vi "FRA-TEC.vi"(0 "LoadProcedure":refnum<k24>, 4 "stop":bool, 7 "error in":errorcluster) -> (18 "Bode phase":cluster{"Y":dbl[], "Y":dbl[]}[](graph), 19 "Bode Z":cluster{"Y":dbl[], "Y":dbl[]}[](graph), 20 "Nyquist":cluster{"Y":dbl[], "Y":dbl[]}[](graph), 21 "E & I":cluster{"Y":dbl[], "Y":dbl[]}[](graph), 22 "-Phase":dbl[](array[numeric]), 23 "Frequency":dbl[](array[numeric]), 24 "-Z''":dbl[](array[numeric]), 25 "Z":dbl[](array[numeric]), 26 "Z'":dbl[](array[numeric]), 27 "error out":errorcluster)   [LabVIEW 2014]
doc: "Shows the Frequency Response Analysis measured values from the instrument."
uses:
  C:/Users/user/Documents/Andre/AutoLAB-2017/Labview/Autolab SDK 1.11/EcoChemie.Autolab.Sdk.dll
  EcoChemie.Autolab.Sdk.dll
  Global 1.vi
  C:/Users/user/Documents/Andre/AutoLAB-2017/Labview/Autolab SDK 1.11/EcoChemie100.dll
  EcoChemie100.dll
panel:
  out "Event":bool
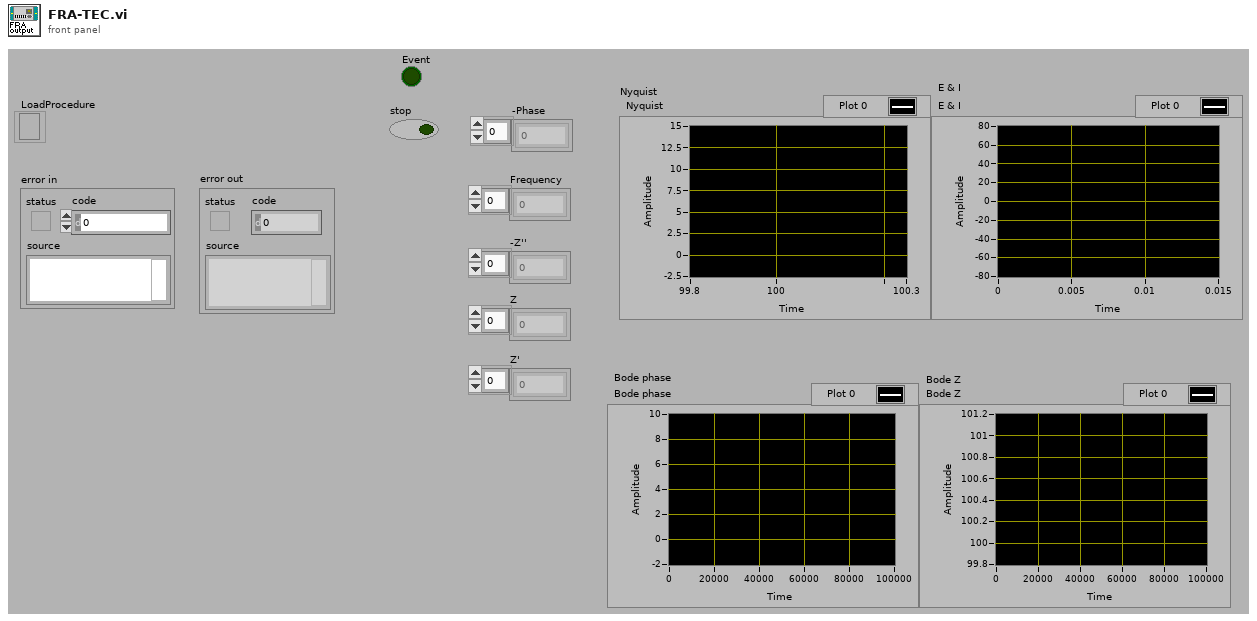
[diagram p1: front panel]
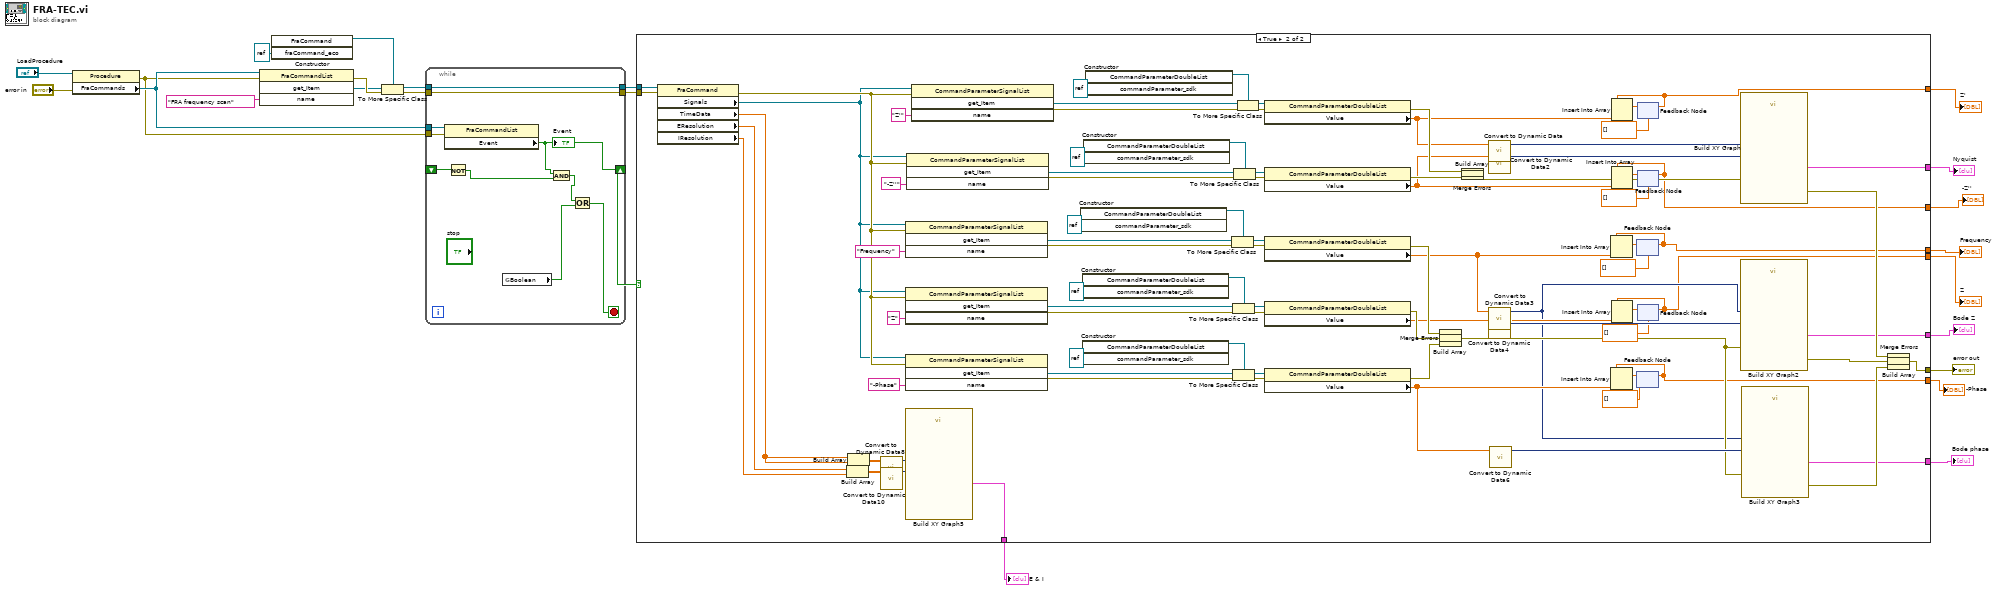
[diagram p0: block diagram]
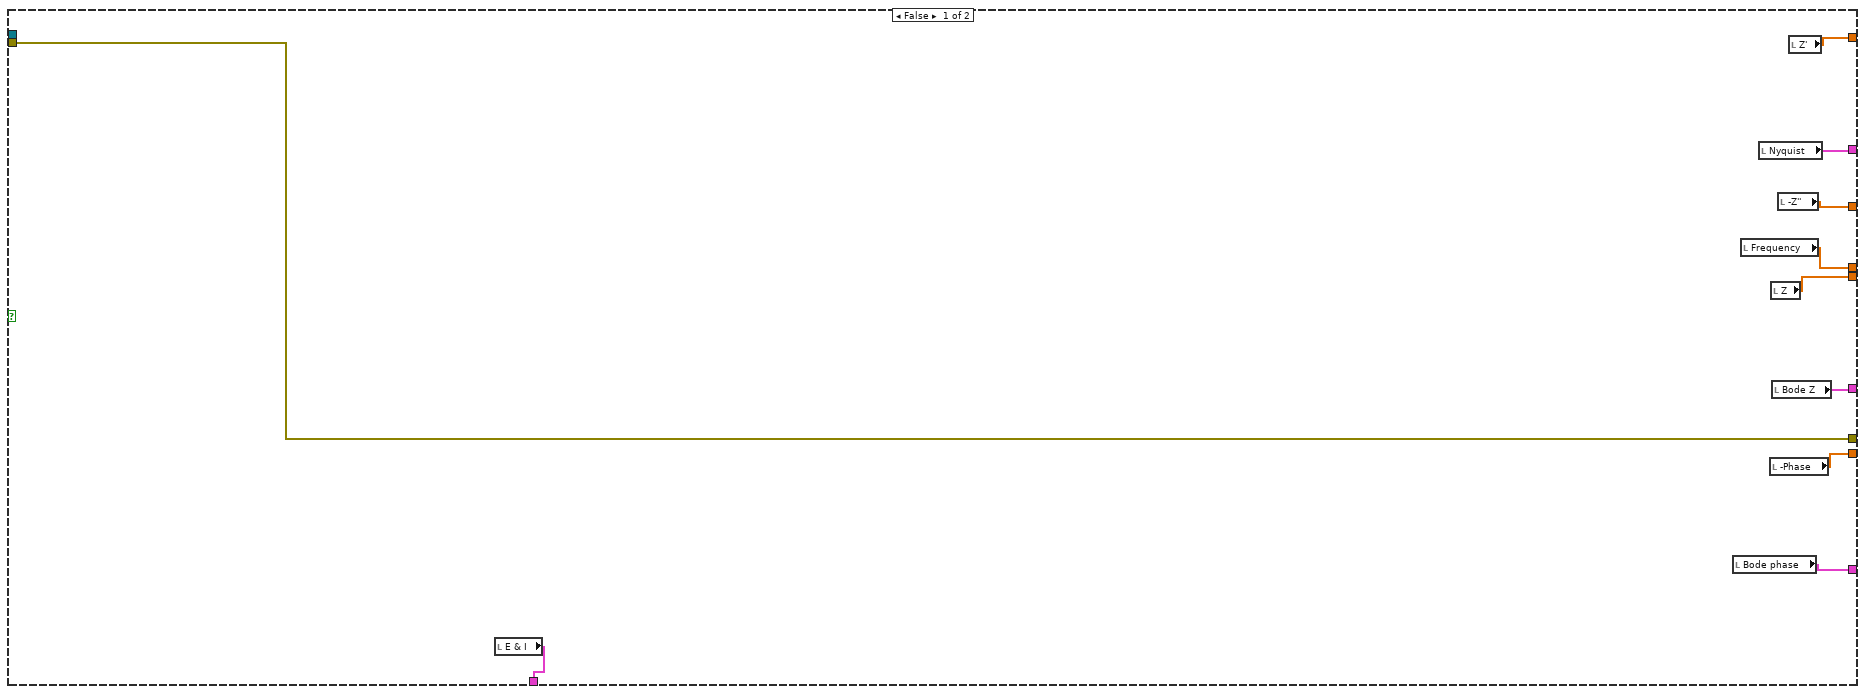
[diagram p2: hidden frame]
diagram:
  n1 = property class="Procedure"(reference="LoadProcedure", error in="error in") -> (error out=w17:errorcluster, "FraCommands"=w18:refnum<k24>)  [unwired: 1 out]
  n2 = invoke class="FraCommandList" method="get_Item"(reference=w18, error in=w17, "name"="FRA frequency scan" ("Fra Commands")) -> (error out=w21:errorcluster, "get_Item"=w20:refnum<k24>)  [unwired: 1 in, 2 out]
  n3 = constructor class="FraCommand"("fraCommand_eco"=refnum<k24> refnum) -> (reference out=w22:refnum<k24>)  [unwired: 3 in, 3 out]
  n4 = To More Specific Class(target class=w22, reference=w20, error in=w21) -> (specific class reference=w3:refnum<k24>, error out=w5:errorcluster)
  n5 = while {
    tunnel: w18 -> [w34]
    tunnel: w17 -> [w33]
    shift-right: [w31] -> w7
    shift-left: _ -> [w32]
    tunnel: [w27] -> w6
    tunnel: w5 -> [w27]
    tunnel: [w26] -> w4
    tunnel: w3 -> [w26]
    stop <- w28 stop-if-true
    n6 = property class="FraCommandList"(reference=w34, error in=w33) -> ("Event"=w31:bool)  [unwired: 2 out]
    "Event" <- w31
    n7 = Not(x=w32) -> (.not. x?=w30:bool)
    n8 = global read "Global 1.vi" "Boolean"() -> (w25:bool)
    n9 = And(x=w31, y=w30) -> (x .and. y?=w29:bool)
    n10 = Or(x=w29, y=w25) -> (x .or. y?=w28:bool)
  }
  n11 = case shown="True" w7 {
    tunnel: [w44 w133] -> w24
    tunnel: w4 -> [_ w132]
    tunnel: w6 -> [w44 w131]
    tunnel: [w40 w61] -> w16
    tunnel: [w41 w60] -> w15
    tunnel: [w42 w59] -> w14
    tunnel: [w43 w58] -> w13
    tunnel: [w35 w57] -> w12
    tunnel: [w36 w56] -> w11
    tunnel: [w37 w55] -> w10
    tunnel: [w38 w54] -> w9
    tunnel: [w39 w53] -> w8
    frame False {
      n12 = local read "E & I"() -> (w43:cluster{"Y":dbl[], "Y":dbl[]}[])
      n13 = local read "Bode phase"() -> (w42:cluster{"Y":dbl[], "Y":dbl[]}[])
      n14 = local read "Frequency"() -> (w37:dbl[])
      n15 = local read "Nyquist"() -> (w40:cluster{"Y":dbl[], "Y":dbl[]}[])
      n16 = local read "-Phase"() -> (w35:dbl[])
      n17 = local read "Z"() -> (w36:dbl[])
      n18 = local read "Bode Z"() -> (w41:cluster{"Y":dbl[], "Y":dbl[]}[])
      n19 = local read "-Z''"() -> (w38:dbl[])
      n20 = local read "Z'"() -> (w39:dbl[])
    }
    frame True {
      n21 = property class="FraCommand"(reference=w132, error in=w131) -> (error out=w105:errorcluster, "Signals"=w104:refnum<k24>, "TimeData"=w65:dbl[], "EResolution"=w64:dbl[], "IResolution"=w63:dbl[])  [unwired: 1 out]
      n22 = Build Array(w64, w63) -> (w90:dbl[][])
      n23 = Build Array(w65, w65) -> (w88:dbl[][])
      n24 = call "Convert to Dynamic Data8"("2D Array"=w88) -> ("Dynamic Data Type"=w87:dynamicdata)  [unwired: 3 in]
      n25 = call "Convert to Dynamic Data10"("2D Array"=w90) -> ("Dynamic Data Type"=w89:dynamicdata)  [unwired: 3 in]
      n26 = invoke class="CommandParameterSignalList" method="get_Item"(reference=w104, error in=w105, "name"="Frequency") -> (error out=w115:errorcluster, "get_Item"=w114:refnum<k24>)  [unwired: 1 in, 2 out]
      n27 = invoke class="CommandParameterSignalList" method="get_Item"(reference=w104, error in=w105, "name"="Z") -> (error out=w120:errorcluster, "get_Item"=w119:refnum<k24>)  [unwired: 1 in, 2 out]
      n28 = invoke class="CommandParameterSignalList" method="get_Item"(reference=w104, error in=w105, "name"="-Phase") -> (error out=w110:errorcluster, "get_Item"=w109:refnum<k24>)  [unwired: 1 in, 2 out]
      n29 = call "Build XY Graph5"("Y Input"=w89, "X Input"=w87) -> ("XY Graph"=w58:cluster{"Y":dbl[], "Y":dbl[]}[])  [unwired: 8 in, 1 out]
      n30 = invoke class="CommandParameterSignalList" method="get_Item"(reference=w104, error in=w105, "name"="-Z''") -> (error out=w130:errorcluster, "get_Item"=w129:refnum<k24>)  [unwired: 1 in, 2 out]
      n31 = invoke class="CommandParameterSignalList" method="get_Item"(reference=w104, error in=w105, "name"="Z'") -> (error out=w125:errorcluster, "get_Item"=w124:refnum<k24>)  [unwired: 1 in, 2 out]
      n32 = constructor class="CommandParameterDoubleList"("commandParameter_sdk"=refnum<k24> refnum) -> (reference out=w113:refnum<k24>)  [unwired: 3 in, 3 out]
      n33 = constructor class="CommandParameterDoubleList"("commandParameter_sdk"=refnum<k24> refnum) -> (reference out=w118:refnum<k24>)  [unwired: 3 in, 3 out]
      n34 = constructor class="CommandParameterDoubleList"("commandParameter_sdk"=refnum<k24> refnum) -> (reference out=w108:refnum<k24>)  [unwired: 3 in, 3 out]
      n35 = constructor class="CommandParameterDoubleList"("commandParameter_sdk"=refnum<k24> refnum) -> (reference out=w128:refnum<k24>)  [unwired: 3 in, 3 out]
      n36 = constructor class="CommandParameterDoubleList"("commandParameter_sdk"=refnum<k24> refnum) -> (reference out=w123:refnum<k24>)  [unwired: 3 in, 3 out]
      n37 = To More Specific Class(target class=w113, reference=w114, error in=w115) -> (specific class reference=w112:refnum<k24>, error out=w111:errorcluster)
      n38 = To More Specific Class(target class=w118, reference=w119, error in=w120) -> (specific class reference=w117:refnum<k24>, error out=w116:errorcluster)
      n39 = To More Specific Class(target class=w108, reference=w109, error in=w110) -> (specific class reference=w107:refnum<k24>, error out=w106:errorcluster)
      n40 = To More Specific Class(target class=w128, reference=w129, error in=w130) -> (specific class reference=w127:refnum<k24>, error out=w126:errorcluster)
      n41 = To More Specific Class(target class=w123, reference=w124, error in=w125) -> (specific class reference=w122:refnum<k24>, error out=w121:errorcluster)
      n42 = property class="CommandParameterDoubleList"(reference=w122, error in=w121) -> (error out=w91:errorcluster, "Value"=w81:dbl[])  [unwired: 1 out]
      n43 = property class="CommandParameterDoubleList"(reference=w127, error in=w126) -> (error out=w92:errorcluster, "Value"=w80:dbl[])  [unwired: 1 out]
      n44 = property class="CommandParameterDoubleList"(reference=w112, error in=w111) -> (error out=w96:errorcluster, "Value"=w84:dbl[])  [unwired: 1 out]
      n45 = property class="CommandParameterDoubleList"(reference=w117, error in=w116) -> (error out=w95:errorcluster, "Value"=w83:dbl[])  [unwired: 1 out]
      n46 = property class="CommandParameterDoubleList"(reference=w107, error in=w106) -> (error out=w94:errorcluster, "Value"=w82:dbl[])  [unwired: 1 out]
      n47 = Build Array(w96, w95, w94) -> (w47:errorcluster[])
      n48 = Merge Errors(w47) -> (w79:errorcluster)
      n49 = Build Array(w91, w92) -> (w46:errorcluster[])
      n50 = Merge Errors(w46) -> (w93:errorcluster)
      n51 = call "Convert to Dynamic Data"("Array"=w81) -> ("Dynamic Data Type"=w98:dynamicdata)  [unwired: 3 in]
      n52 = call "Convert to Dynamic Data2"("Array"=w80) -> ("Dynamic Data Type"=w97:dynamicdata)  [unwired: 3 in]
      n53 = call "Convert to Dynamic Data3"("Array"=w84) -> ("Dynamic Data Type"=w62:dynamicdata)  [unwired: 3 in]
      n54 = call "Convert to Dynamic Data4"("Array"=w83) -> ("Dynamic Data Type"=w86:dynamicdata)  [unwired: 3 in]
      n55 = call "Convert to Dynamic Data6"("Array"=w82) -> ("Dynamic Data Type"=w85:dynamicdata)  [unwired: 3 in]
      n56 = feedback #1(dbl[] []) -> (w55:dbl[])
      n57 = Insert Into Array(array=w55, new element=w84) -> (w75:dbl[])  [unwired: 1 in]
      n58 = feedback-in #1(w75) -> ()
      n59 = feedback #2(dbl[] []) -> (w57:dbl[])
      n60 = Insert Into Array(array=w57, new element=w82) -> (w73:dbl[])  [unwired: 1 in]
      n61 = feedback-in #2(w73) -> ()
      n62 = feedback #3(dbl[] []) -> (w53:dbl[])
      n63 = Insert Into Array(array=w53, new element=w81) -> (w72:dbl[])  [unwired: 1 in]
      n64 = feedback-in #3(w72) -> ()
      n65 = feedback #4(dbl[] []) -> (w54:dbl[])
      n66 = Insert Into Array(array=w54, new element=w80) -> (w71:dbl[])  [unwired: 1 in]
      n67 = feedback-in #4(w71) -> ()
      n68 = feedback #5(dbl[] []) -> (w56:dbl[])
      n69 = Insert Into Array(array=w56, new element=w83) -> (w74:dbl[])  [unwired: 1 in]
      n70 = feedback-in #5(w74) -> ()
      n71 = call "Build XY Graph"("error in (no error)"=w93, "Y Input"=w97, "X Input"=w98) -> ("error out"=w77:errorcluster, "XY Graph"=w61:cluster{"Y":dbl[], "Y":dbl[]}[])  [unwired: 7 in]
      n72 = call "Build XY Graph2"("error in (no error)"=w79, "Y Input"=w86, "X Input"=w62) -> ("error out"=w78:errorcluster, "XY Graph"=w60:cluster{"Y":dbl[], "Y":dbl[]}[])  [unwired: 7 in]
      n73 = call "Build XY Graph3"("error in (no error)"=w79, "Y Input"=w85, "X Input"=w62) -> ("error out"=w76:errorcluster, "XY Graph"=w59:cluster{"Y":dbl[], "Y":dbl[]}[])  [unwired: 7 in]
      n74 = Build Array(w77, w78, w76) -> (w45:errorcluster[])
      n75 = Merge Errors(w45) -> (w133:errorcluster)
    }
  }
  "error out" <- w24
  "Nyquist" <- w16
  "Bode Z" <- w15
  "Bode phase" <- w14
  "E & I" <- w13
  "Z'" <- w8
  "-Z''" <- w9
  "Frequency" <- w10
  "Z" <- w11
  "-Phase" <- w12
